vi "Configure Measurement.vi"(8 "error in (no error)":errorcluster, 10 "Meas Setting":T1={"Function (0: DC Voltage)"=0, "Manual Resolution (5.5 Digits)"=5.5, "Manual Range (1.00)"=1.0, "Enable Auto Range (T: Enable)"=TRUE} {"Manual Range (1.00)" format="%_3f"; "Manual Resolution (5.5 Digits)" items=["4.5"=4.5, "5.5"=5.5, "6.5"=6.5]; "Function (0: DC Voltage)" items=["DC Voltage", "AC Voltage", "2 - Wire Resistance", "4 - Wire Resistance", "DC Current", "AC Current", "Frequency", "Period", "Continuity", "Diode Checking", "VDC:VDC Ratio", "Temperature", "Capacitance"]}, 11 "Agilent 34401A in":refnum<class "Agilent 34401A.lvclass">) -> (0 "error out":errorcluster, 3 "Agilent 34401A out":refnum<class "Agilent 34401A.lvclass">)   [LabVIEW 2016, in "DMM.lvlib" / "Agilent 34401A.lvclass"]
uses:
  Agilent 34401A.lvclass
  Agilent 34401A.lvclass/Agilent 34401A.ctl
  <instrlib>/Agilent 34401/Agilent 34401.lvlib
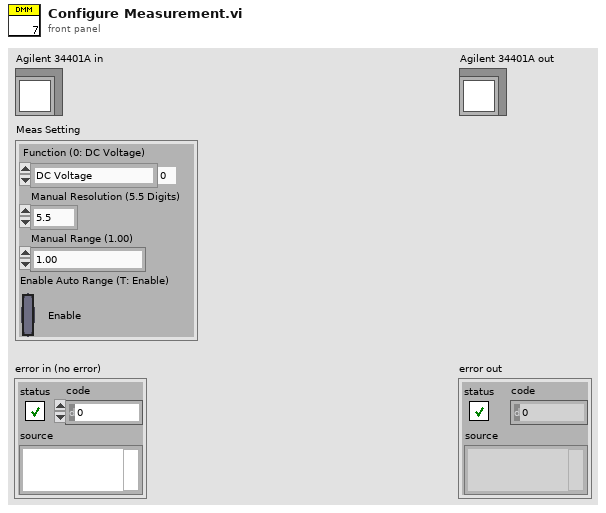
[diagram p1: front panel]
types:
  T1 = cluster{"Function (0: DC Voltage)":u16, "Manual Resolution (5.5 Digits)":dbl, "Manual Range (1.00)":dbl, "Enable Auto Range (T: Enable)":bool}
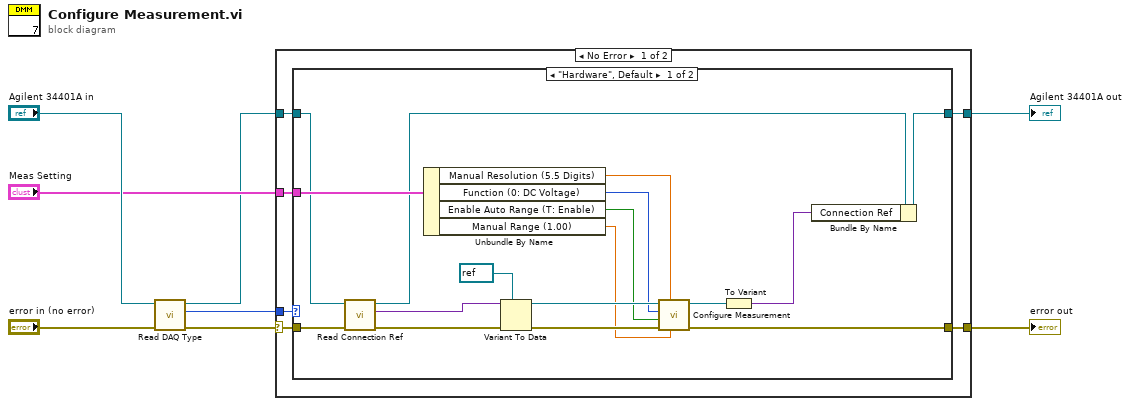
[diagram p0: block diagram]
diagram:
  n1 = call-dynamic "Read DAQ Type.vi"("error in (no error)"="error in (no error)", "Agilent 34401A in"="Agilent 34401A in") -> ("error out"=w7:errorcluster, "DAQ Type"=w6:enum16{"Hardware", "Simulation"}, "Agilent 34401A out"=w1:refnum<class "Agilent 34401A.lvclass">)  [unwired: 7 in]
  n2 = case shown="No Error" w7 {
    selector: w7 -> [w11 w34]
    tunnel: w6 -> [w14 _]
    tunnel: w1 -> [w13 w35]
    tunnel: [w12 w35] -> w4
    tunnel: [w10 w34] -> w3
    tunnel: "Meas Setting" -> [w9 _]
    frame No Error {
      n3 = case shown="\"Hardware\", Default" w14 {
        tunnel: w13 -> [w16 w33]
        tunnel: [w19 w33] -> w12
        tunnel: w11 -> [w31 w32]
        tunnel: [w27 w32] -> w10
        tunnel: w9 -> [w24 _]
        frame "Hardware", Default {
          n4 = call-dynamic "Read Connection Ref.vi"("error in (no error)"=w31, "Agilent 34401A in"=w16) -> ("error out"=w30:errorcluster, "Connection Ref"=w29:variant, "Agilent 34401A out"=w15:refnum<class "Agilent 34401A.lvclass">)  [unwired: 7 in]
          n5 = Unbundle By Name(w24) -> ("Manual Resolution (5.5 Digits)"=w22:dbl, "Function (0: DC Voltage)"=w23:u16, "Enable Auto Range (T: Enable)"=w21:bool, "Manual Range (1.00)"=w20:dbl)
          n6 = Variant To Data(error in=w30, type=refnum<visa-resource-name> refnum ("VISA resource name"), Variant=w29) -> (data=w25:refnum<visa-resource-name>, error out=w28:errorcluster)
          n7 = call <instrlib>:"Configure Measurement.vi"("Manual Range (1.00)"=w20, "Manual Resolution (5.5 Digits)"=w22, "error in (no error)"=w28, "Enable Auto Range (T: Enable)"=w21, "Function (0: DC Voltage)"=w23, "VISA resource name"=w25) -> ("error out"=w27:errorcluster, "VISA resource name out"=w18:refnum<visa-resource-name>)  [unwired: 4 in]
          n8 = To Variant(anything=w18) -> (Variant=w17:variant)
          n9 = Bundle By Name(cluster=w15, "Connection Ref"=w17) -> (w19:refnum<class "Agilent 34401A.lvclass">)
        }
        frame "Simulation" {
        }
      }
    }
    frame Error {
    }
  }
  "error out" <- w3
  "Agilent 34401A out" <- w4
